vi "quaternion_conjugate.vi"(11 "Q":dbl[](array[numeric])) -> (3 "Q conjugate":dbl[](array[numeric]))   [LabVIEW 2012]
panel:
  # "For unit quaternions, the conjugate is the inverse."
  # "w"
  # "x1"
  # "x2"
  # "x3"
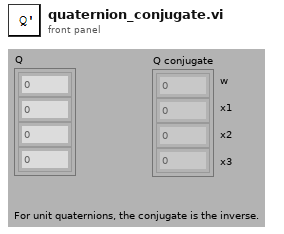
[diagram p1: front panel]
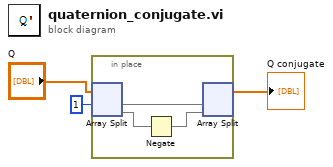
[diagram p0: block diagram]
diagram:
  n1 = in-place {
    n2 = in-place-split #1("Q", 1) -> (w6:dbl[], w5:dbl[])
    n3 = Negate(x=w5) -> (-x=w4:dbl[])
    n4 = in-place-split #1(w6, w4) -> (→"Q conjugate":dbl[])  [unwired: 1 out]
  }
